vi "Simple_Add.vi"() -> ()   [LabVIEW 2018]
panel:
  in  "z":dbl
  out "sum":dbl
  in  "x":dbl
  in  "y":dbl
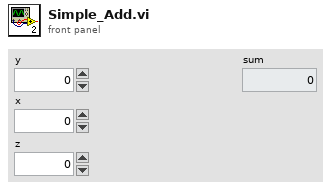
[diagram p1: front panel]
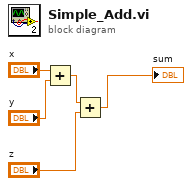
[diagram p0: block diagram]
diagram:
  n1 = Add(x="x", y="y") -> (x+y=w3:dbl)
  n2 = Add(x=w3, y="z") -> (x+y=→"sum":dbl)
